vi "P2-1.vi"() -> ()   [LabVIEW 2011]
panel:
  out "불리언":bool
  in  "숫자형 2":dbl
  in  "숫자형":dbl
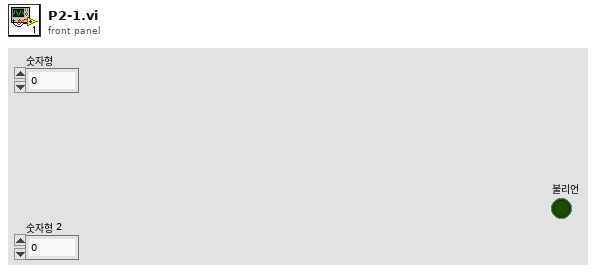
[diagram p1: front panel]
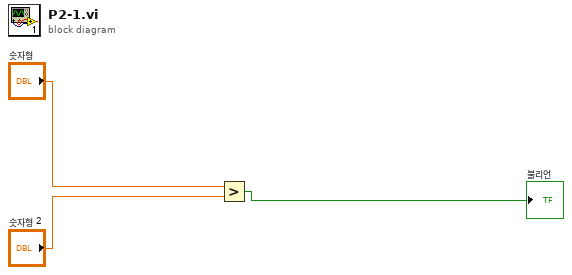
[diagram p0: block diagram]
diagram:
  n1 = Greater?(x="숫자형", y="숫자형 2") -> (0:→"불리언":bool)
